vi "LIDAR V9 FPGA Main.vi"() -> ()   [LabVIEW 2013]
uses:
  Controls/FPGA Nain State.ctl
  Controls/Scan Format Typedaf.ctl
  <vilib>/Platform/TimedLoop/XDataNode/timing_clust.ctl
  <vilib>/Platform/TimedLoop/XDataNode/nitl_modes.ctl
  <vilib>/Platform/TimedLoop/XDataNode/wakeup.ctl
  Controls/Algorithm State.ctl
  <vilib>/rvi/Emulation/niFpgaSctlEmulationGetInTimedLoop.vi
  <vilib>/rvi/DataTransferAndStorage/Container/Common/niFpgaContainerGetUniqueNameForEmu.vi
  <vilib>/rvi/DataTransferAndStorage/Container/Common/niFpgaContainerSetEmuInfo.vi
  <vilib>/rvi/eio/common/nirviEmuReportErrorAndStop.vi
  <vilib>/rvi/Emulation/niFpgaEmulationReportErrorSimple.vi
  <vilib>/rvi/Emulation/niFpgaGetClockAttributes.vi
  <vilib>/rvi/Emulation/niFpgaCriticalErrorInLSC.vi
  <vilib>/rvi/eio/common/nirviEmuTemplateMethod_errors.vi
  <vilib>/rvi/FIFO/Fifo_Resource/nirvififoEmulationWriteFpgaImpl.vi
  <vilib>/rvi/DataTransferAndStorage/Container/Common/niFpgaContainerExecOnDevCompGetState.vi
  <vilib>/rvi/DataTransferAndStorage/Register/Emulation/niFpgaRegisterEmulationFpgaImpl.vi
  <instcachedir>/0/niFpgaRegisterEmulationFpgaImpl_DCF4BC0110594B98B44A971D60CEEC4D.lvgen/niFpgaRegisterEmulationFpgaImpl_DCF4BC0110594B98B44A971D60CEEC4D_000.vi
  <vilib>/rvi/FIFO/Fifo_Resource/nirvififoEmulationReadFpgaImpl.vi
  LIDAR V2 Globals.vi
  <vilib>/rvi/Emulation/niFpgaProcessEmulError.vi
  <vilib>/rvi/interface/RandomDataEmulation/nirviRandomDataFPGAFIFO.vi
  <vilib>/rvi/interface/RandomDataEmulation/niFpgaRandomDataHandleErrors.vi
  <vilib>/Platform/TimedLoop/XDataNode/XDataNode.xnode
  <vilib>/rvi/LocalResourceManager/LocalResourceManager.xnode
  <vilib>/eio/EIONode/EIONode.xnode
  <vilib>/rvi/DataTransferAndStorage/Container/XNode/niFpgaContainer.xnode
  <vilib>/rvi/FIFO/Fifo_Resource/nirvififoEmulationWrite.vi
  <vilib>/rvi/DataTransferAndStorage/Register/Emulation/niFpgaRegisterEmulationRefIn.vi
  <vilib>/rvi/FIFO/Fifo_Resource/nirvififoEmulationRead.vi
  <vilib>/rvi/interface/RandomDataEmulation/nirviRandomDataFpgaReadWriteTemplate.vi
  <vilib>/Platform/TimedLoop/XDataNode/XDNodeRunTimeDep.lvlib
panel:
  in  "MaxStartSample":u8
  in  "LedScanDebEn":bool
  in  "ActiveLedIndexDeb":u16
  in  "10thIndexDeb":u8
  in  "PulseUpClck":u16=3
  in  "PulseWaitClck":u16=40
  in  "Devider":u8=3
  in  "PFI3":bool
  in  "PFI2":bool
  in  "User Command Commit":bool
  in  "User Command":u8
  out "User Command Idle":bool
  out "User Command Status":u8
  in  "User Data 0":u8
  in  "User Data 1":u8
  out "User Error":bool
  out "Configured?":bool
  in  "MemDebStart":u32
  in  "MemDebEnd":u32
  in  "ReadMemSel":bool
  in  "ReadMem":bool
  in  "NextLedEn":bool
  out "SimOut":i16
  out "PLL Locked":bool
  out "LedAddress":u16
  in  "SingleCycle":bool
  in  "PulsePerLed":i16=199
  in  "ScanFormat":T1=enum."FullScanPerLed"
  in  "SamplingEnable":bool
  out "MainState":T2
  out "10thIndex":u8
  out "PulseIndex":i16
  in  "MemSel":bool
  in  "ActiveLedIndex":u16
  out "InitMem":bool
  out "PulseEnd":bool
  in  "SampPerPulse":u16=99
  out "IterReset":u16 format="%.0b"
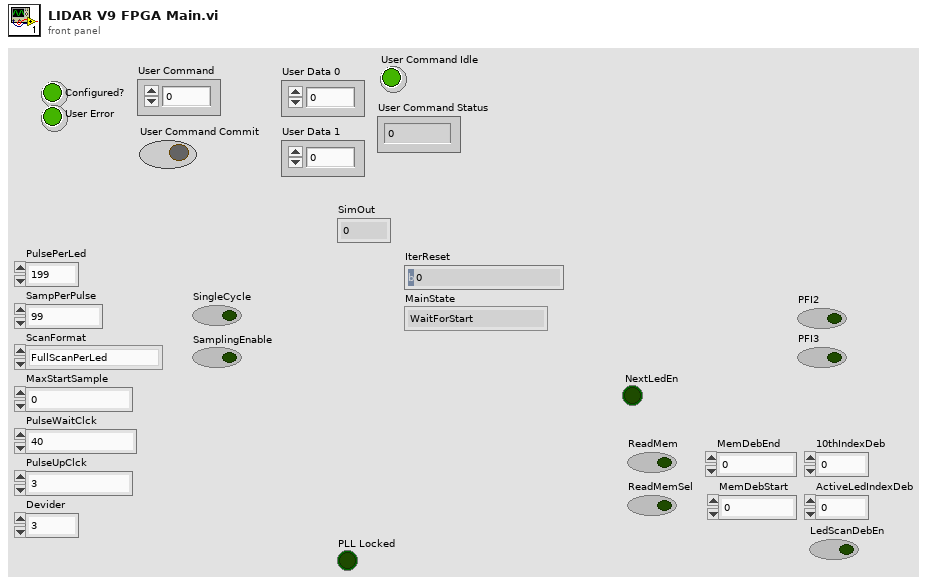
[diagram p1: front panel]
types:
  T1 = typedef "Scan Format Typedaf.ctl" = enum16{"1PulsePerLed", "FullScanPerLed"}
  T2 = typedef "FPGA Nain State.ctl" = enum16{"WaitForStart", "SetProcParams", "SelectActiveLed", "ActivatePulse", "WaitForPulseEnd", "WaitForAlgoStart", "SingleCycleEnd"}
  T3 = typedef "XDNodeRunTimeDep.lvlib/timing_clust.ctl" = cluster{"Expected End [f-1]":u64, "Actual End [f-1]":u64, "Finished Late? [f-1]":bool, "Expected End [i-1]":u64, "Actual End [i-1]":u64, "Finished Late? [i-1]":bool, "Expected Start [i]":u64, "Actual Start [i]":u64, "Expected Start [f]":u64, "Actual Start [f]":u64, "Source Name":string, "Structure Name":string, "Period":i64, "Deadline":i64, "Offset":i64, "Start":i64, "Priority":i32, "Timeout":i32, "Mode":T4, "Wakeup Reason":T5, "Error":errorcluster, "Source Type":string, "Secondary Source Type":string, "Global End Time":u64, "Global Start Time":u64, "Frame Duration":u64, "Iteration Duration":u64, "Assigned CPU":i32, "I/O Scan Engine Mode":u32}
  T4 = typedef "XDNodeRunTimeDep.lvlib/nitl_modes.ctl" = enum32{"No Change", "Process missed periods, maintain original phase", "Discard missed periods, maintain original phase", "Process missed periods, ignore original phase", "Discard missed periods, ignore original phase"}
  T5 = typedef "XDNodeRunTimeDep.lvlib/wakeup.ctl" = enum32{"Normal", "Aborted", "Asynchronous wakeup", "Timing source error", "Timed loop error", "Timeout"}
  T6 = typedef "Algorithm State.ctl" = enum16{"WaitForStart", "GetNextSignalElement", "WaitForNextSignalElem", "MultWithSinc", "CalcMax"}
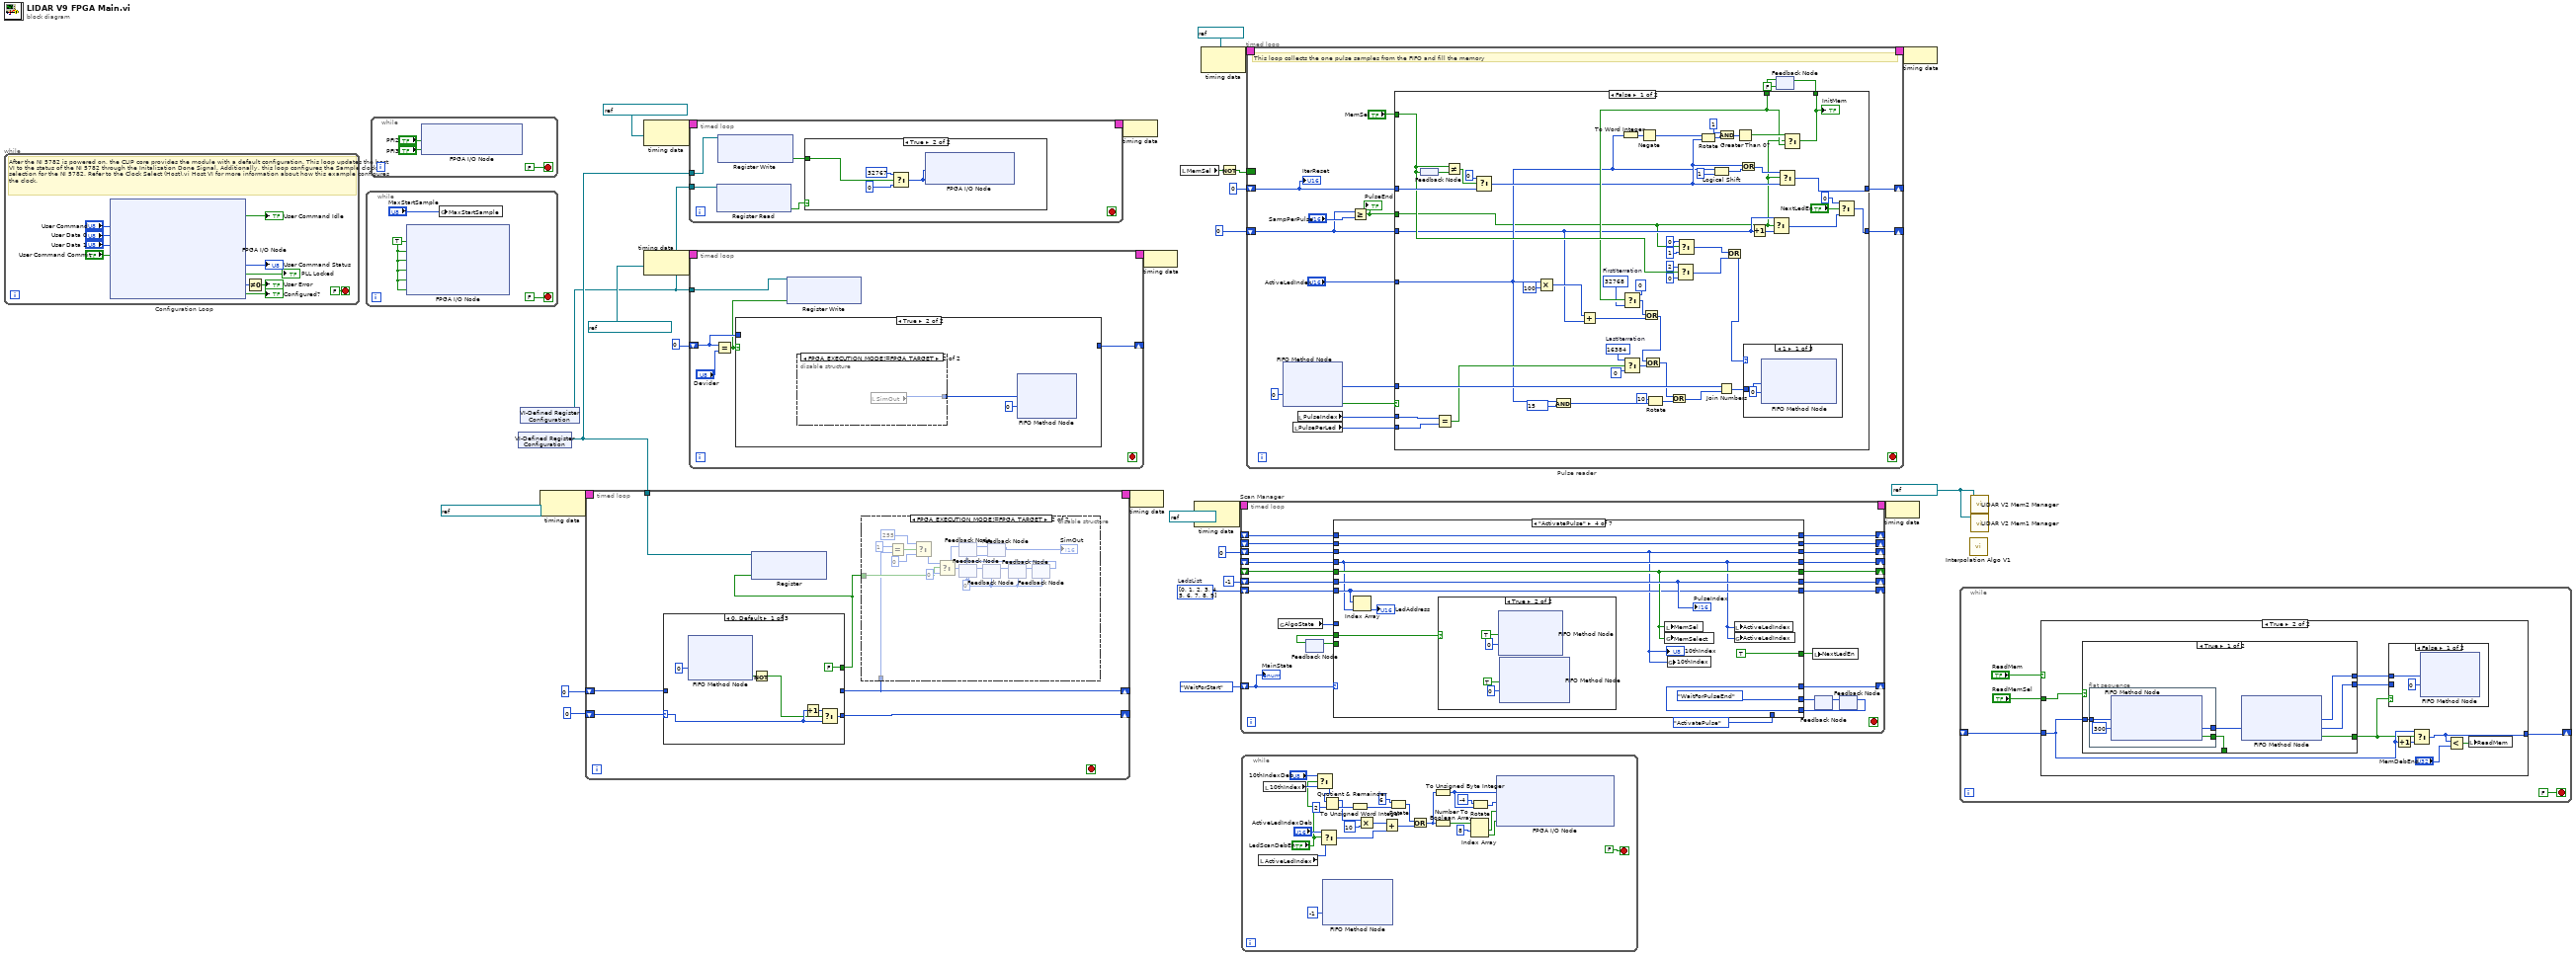
[diagram p0: block diagram]
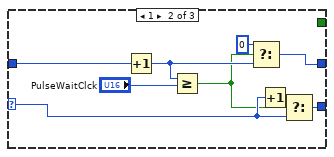
[diagram p4: hidden frame]
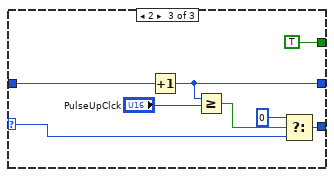
[diagram p5: hidden frame]
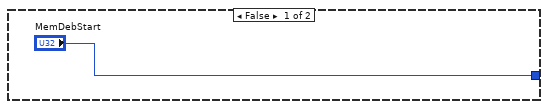
[diagram p6: hidden frame]
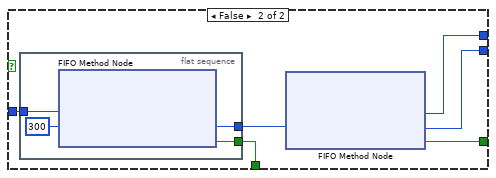
[diagram p8: hidden frame]
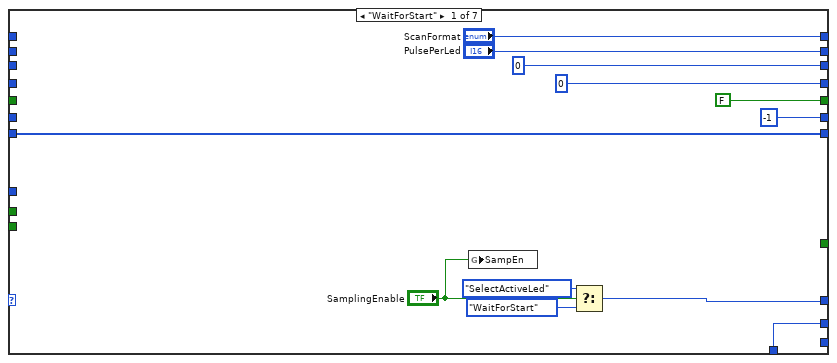
[diagram p9: hidden frame]
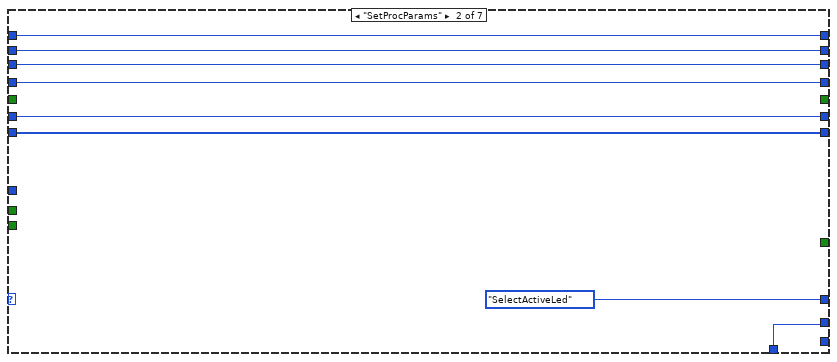
[diagram p10: hidden frame]
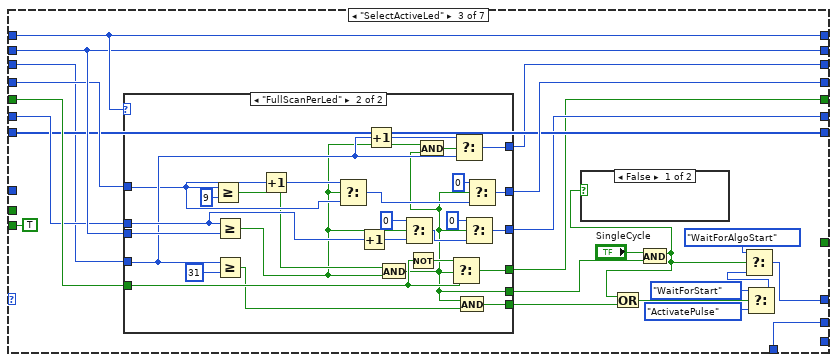
[diagram p11: hidden frame]
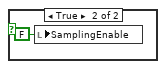
[diagram p12: hidden frame]
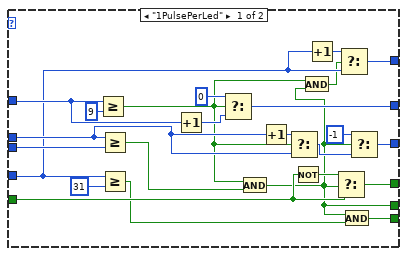
[diagram p13: hidden frame]
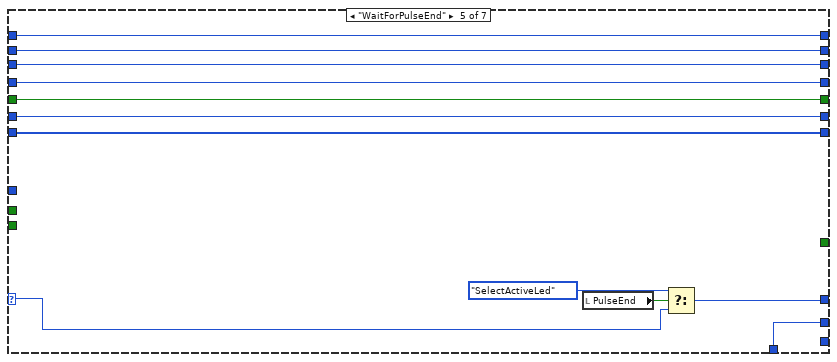
[diagram p15: hidden frame]
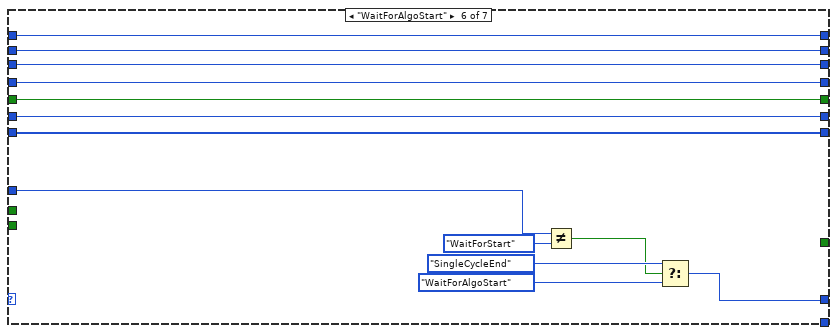
[diagram p16: hidden frame]
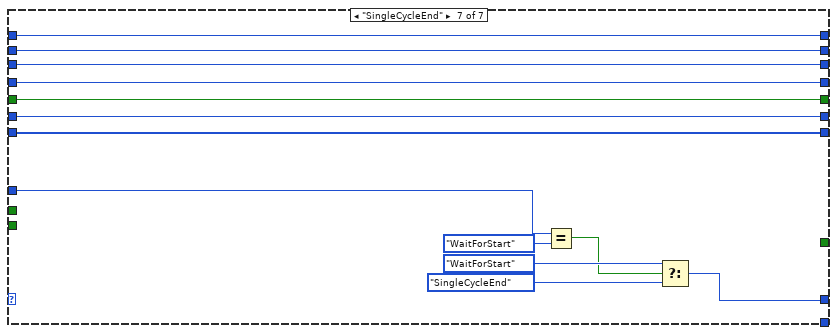
[diagram p17: hidden frame]
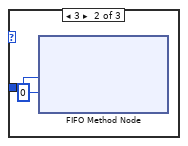
[diagram p18: hidden frame]
diagram:
  w1 = refnum<k21> "83.33MHz" ("Source Name")
  w17 = u16[] [0, 1, 2, 3, 4, 5, 6, 7, 8, 9]  # LedsList
  n1 = while "Configuration Loop" {
    stop <- FALSE stop-if-true
    # "After the NI 5782 is powered on, the CLIP core provides the module with a default configuration. This loop updates the host VI to the status of the NI 5782 through the Initalization Done Signal. Additionally, this loop configures the Sample clock selection for the NI 5782. Refer to the Clock Select (Host).vi Host VI for more information about how this example configures the clock."
    n2 = xnode "FPGA I/O Node"("IO Module\\User Command"="User Command", "IO Module\\User Data 0"="User Data 0", "IO Module\\User Data 1"="User Data 1", "IO Module\\User Command Commit"="User Command Commit") -> ("IO Module\\User Command Idle"=→"User Command Idle":bool, "IO Module\\User Command Status"=→"User Command Status":u8, "IO Module\\PLL Locked"=→"PLL Locked":bool, "IO Module\\User Error"=w34:u8, "IO Module\\Initialization Done"=→"Configured?":bool)  [unwired: 9 in, 9 out]
    n3 = Not Equal To 0?(x=w34) -> (x != 0?=→"User Error":bool)
  }
  n4 = while {
    stop <- FALSE stop-if-true
    w42 = TRUE ("IO Module\\DIO Port 0 WE")
    n5 = xnode "FPGA I/O Node"("IO Module\\DIO Port 0 WE"=w42, "IO Module\\DIO Port 1 WE"=w42, "IO Module\\PFI 0 WE"=w42, "IO Module\\PFI 1 WE"=w42, "IO Module\\PFI 2 WE"=w42, "IO Module\\PFI 3 WE"=w42) -> ()  [unwired: 6 in, 6 out]
    n6 = global write "LIDAR V2 Globals.vi" "MaxStartSample"("MaxStartSample") -> ()
  }
  n7 = while {
    stop <- FALSE stop-if-true
    n8 = xnode "FPGA I/O Node"("IO Module\\PFI 2 Wr Data"="PFI2", "IO Module\\PFI 3 Wr Data"="PFI3") -> ()  [unwired: 2 in, 2 out]
  }
  n9 = xnode ("VI-Defined Register Configuration")() -> ("Register Out"=w3:refnum<k21>)
  n10 = xnode ("VI-Defined Register Configuration")() -> ("Register Out"=w2:refnum<k21>)
  n11 = node-c288(refnum<k21> "IO Module\\Data Clock Div 2" ("Source Name")) -> (w11:T3)
  n12 = timed-loop {
    timing: w11 -> [_]
    timing-out: [_] -> w10
    shift-right: [w51] -> _
    shift-left: i16 0 -> [w52]
    shift-right: [w49] -> _
    shift-left: u16 0 -> [w50]
    tunnel: w3 -> [w48]
    stop <- _ stop-if-true
    n13 = case shown="0, Default" w52 {
      selector: w52 -> [w74 w81 w87]
      tunnel: [w75 w82 w88] -> w51
      tunnel: w50 -> [_ w84 w92]
      tunnel: [_ w78 w91] -> w49
      tunnel: [FALSE _ TRUE] -> w47
      frame 0, Default {
        n14 = xnode ("FIFO Method Node")("Timeout"=0) -> ("Timed Out?"=w71:bool)  [unwired: 1 in, 2 out]
        n15 = Not(x=w71) -> (.not. x?=w69:bool)
        n16 = Increment(x=w74) -> (x+1=w73:i16)
        n17 = Select(t=w73, s=w69, f=w74) -> (s? t:f=w75:i16)
      }
      frame 1 {
        n18 = Increment(x=w84) -> (x+1=w79:u16)
        n19 = Greater Or Equal?(x=w79, y="PulseWaitClck") -> (x >= y?=w76:bool)
        n20 = Select(t=u16 0, s=w76, f=w79) -> (s? t:f=w78:u16)
        n21 = Increment(x=w81) -> (x+1=w80:i16)
        n22 = Select(t=w80, s=w76, f=w81) -> (s? t:f=w82:i16)
      }
      frame 2 {
        n23 = Increment(x=w92) -> (x+1=w91:u16)
        n24 = Greater Or Equal?(x=w91, y="PulseUpClck") -> (x >= y?=w89:bool)
        n25 = Select(t=i16 0, s=w89, f=w87) -> (s? t:f=w88:i16)
      }
    }
    n26 = xnode "Register"("Data"=w47, "Register In"=w48) -> ()  [unwired: 1 out]
    n27 = disable-structure shown="FPGA_EXECUTION_MODE!=FPGA_TARGET" {
      disable-tunnel: w47 -> [_ w60]
      disable-tunnel: w49 -> [_ w59]
      frame condition #0 (active) {
      }
      frame condition #1 {
        w63 = i16 0 ("IO Module\\AO 0")
        n28 = Equal?(x=u16 1, y=w59) -> (x = y?=w57:bool)
        n29 = Select(t=i16 255 ("IO Module\\AO 0"), s=w57, f=i16 0) -> (s? t:f=w58:i16)
        n30 = Select(t=w58, s=w60, f=i16 0 ("IO Module\\AO 0")) -> (s? t:f=w61:i16)
        n31 = feedback-in #1(w61) -> ()
        n32 = feedback #1(w63) -> (w68:i16)
        n33 = feedback #2(w63) -> (w64:i16)
        n34 = feedback #3(w63) -> (w67:i16)
        n35 = feedback-in #3(w68) -> ()
        n36 = feedback #4(w63) -> (→"SimOut":i16)
        n37 = feedback-in #4(w64) -> ()
        n38 = feedback #5(w63) -> (w66:i16)
        n39 = feedback-in #5(w67) -> ()
        n40 = feedback #6(w63) -> (w65:i16)
        n41 = feedback-in #2(w65) -> ()
        n42 = feedback-in #6(w66) -> ()
      }
    }
  }
  n43 = node-c288(refnum<k21> "IO Module\\Data Clock" ("Source Name")) -> (w6:T3)
  n44 = node-c288(refnum<k21> "IO Module\\Data Clock" ("Source Name")) -> (w29:T3)
  n45 = timed-loop {
    timing: w6 -> [_]
    timing-out: [_] -> w5
    tunnel: w3 -> [w98]
    tunnel: w2 -> [w96]
    stop <- _ stop-if-true
    n46 = xnode "Register Read"("Register In"=w96) -> ("Data"=w95:bool)  [unwired: 1 out]
    n47 = xnode "Register Write"("Register In"=w98) -> ("Data"=w97:bool)  [unwired: 1 out]
    n48 = case shown="True" w95 {
      tunnel: w97 -> [_ w99]
      frame False {
      }
      frame True {
        n49 = Select(t=i16 32767 ("IO Module\\AO 0"), s=w99, f=i16 0 ("IO Module\\AO 0")) -> (s? t:f=w100:i16)
        n50 = xnode "FPGA I/O Node"("IO Module\\AO 0 N-1"=w100, "IO Module\\AO 0 N"=w100) -> ()  [unwired: 2 in, 2 out]
      }
    }
  }
  n51 = timed-loop {
    timing: w29 -> [_]
    timing-out: [_] -> w28
    shift-right: [w107] -> _
    shift-left: u8 0 -> [w108]
    tunnel: w2 -> [w106]
    stop <- _ stop-if-true
    n52 = Equal?(x=w108, y="Devider") -> (x = y?=w105:bool)
    n53 = case shown="True" w105 {
      tunnel: w108 -> [w111 _]
      tunnel: [w110 _] -> w107
      frame False {
        n54 = Increment(x=w111) -> (x+1=w110:u8)
      }
      frame True {
        n55 = disable-structure shown="FPGA_EXECUTION_MODE!=FPGA_TARGET" {
          disable-tunnel: [w114 w115] -> w112
          frame condition #0 (active) {
            n56 = xnode "FPGA I/O Node"() -> ("IO Module\\AI 0"=w114:i16)  [unwired: 1 in, 1 out]
          }
          frame condition #1 {
            n57 = local read "SimOut"() -> (w115:i16)
          }
        }
        n58 = xnode ("FIFO Method Node")("Element"=w112, "Timeout"=0) -> ()  [unwired: 1 in, 2 out]
      }
    }
    n59 = xnode "Register Write"("Data"=w105, "Register In"=w106) -> ()  [unwired: 1 out]
  }
  n60 = node-c288(w5) -> ()
  n61 = node-c288(w10) -> ()
  n62 = node-c288(w28) -> ()
  n63 = local read "MemSel"() -> (w22:bool)
  n64 = node-c288(refnum<k21> "83.33MHz" ("Source Name")) -> (w25:T3)
  n65 = node-c288(refnum<k21> "83.33MHz" ("Source Name")) -> (w27:T3)
  n66 = Not(x=w22) -> (.not. x?=w21:bool)
  n67 = timed-loop "Scan Manager" {
    timing: w25 -> [_]
    timing-out: [_] -> w24
    shift-right: [w140] -> _
    shift-left: FPGA_Nain_State."WaitForStart" ("MainState") -> [w141]
    shift-right: [w139] -> _
    shift-left: _ -> [w137]
    shift-right: [w138] -> _
    shift-left: _ -> [w136]
    shift-right: [w129] -> _
    shift-left: u8 0 ("10thIndex") -> [w135]
    shift-right: [w119] -> _
    shift-left: _ -> [w134]
    shift-right: [w123] -> _
    shift-left: _ -> [w133]
    shift-right: [w132] -> _
    shift-left: i16 -1 -> [w122]
    shift-right: [w130] -> _
    shift-left: w17 -> [w131]
    stop <- _ stop-if-true
    n68 = global read "LIDAR V2 Globals.vi" "AlgoState"() -> (w118:T6)
    n69 = feedback #7() -> (w120:bool)  [unwired: 1 in]
    n70 = feedback #8() -> (w126:T2)  [unwired: 1 in]
    n71 = feedback #9() -> (w125:T2)  [unwired: 1 in]
    n72 = case shown="\"ActivatePulse\"" w141 {
      selector: w141 -> [_ _ _ _ w257 _ _]
      tunnel: [w151 FPGA_Nain_State."SelectActiveLed" ("MainState") w165 w243 w256 w267 w280] -> w140
      tunnel: ["ScanFormat" w157 w184 w247 w263 w276 w289] -> w139
      tunnel: ["PulsePerLed" w156 w182 w246 w262 w275 w288] -> w138
      tunnel: w137 -> [_ w157 w184 w247 w263 w276 w289]
      tunnel: w136 -> [_ w156 w182 w246 w262 w275 w288]
      tunnel: [u8 0 ("10thIndex") w155 w173 w236 w261 w274 w287] -> w129
      tunnel: w135 -> [_ w155 w174 w236 w261 w274 w287]
      tunnel: [u16 0 ("ActiveLedIndex") w154 w179 w237 w260 w273 w286] -> w119
      tunnel: w134 -> [_ w154 w180 w237 w260 w273 w286]
      tunnel: [FALSE _ w176 w240 w259 w272 w285] -> w123
      tunnel: w133 -> [_ _ w183 w240 w259 w272 w285]
      tunnel: [i16 -1 ("t") w160 w177 w241 w254 w271 w284] -> w132
      tunnel: w122 -> [_ w160 w181 w241 w254 w271 w284]
      tunnel: w131 -> [w149 w159 w178 w238 w253 w270 w283]
      tunnel: [w149 w159 w178 w238 w253 w270 w283] -> w130
      tunnel: [_ _ _ TRUE ("SampEnable") _ _ _] -> w128
      tunnel: [w148 w158 w172 FPGA_Nain_State."WaitForPulseEnd" ("MainState") w252 _ _] -> w127
      tunnel: w125 -> [_ _ _ w243 _ _ _]
      tunnel: FPGA_Nain_State."ActivatePulse" ("MainState") -> [w148 w158 w172 _ w252 _ _]
      tunnel: [_ _ TRUE _ _ _ _] -> w121
      tunnel: w120 -> [_ _ _ w242 _ _ _]
      tunnel: w118 -> [_ _ _ _ _ w264 w278]
      frame "WaitForStart" {
        n73 = global write "LIDAR V2 Globals.vi" "SampEn"("SamplingEnable") -> ()
        n74 = Select(t=FPGA_Nain_State."SelectActiveLed" ("MainState"), s="SamplingEnable", f=FPGA_Nain_State."WaitForStart" ("MainState")) -> (s? t:f=w151:T2)
      }
      frame "SetProcParams" {
      }
      frame "SelectActiveLed" {
        n75 = case shown="\"FullScanPerLed\"" w184 {
          tunnel: w183 -> [w201 w231]
          tunnel: w174 -> [w194 w226]
          tunnel: w182 -> [w204 w233]
          tunnel: w180 -> [w207 w217]
          tunnel: w181 -> [w203 w232]
          tunnel: [w195 w213] -> w179
          tunnel: [w190 w215] -> w177
          tunnel: [w198 w229] -> w176
          tunnel: [w196 w227] -> w170
          tunnel: [w192 w224] -> w173
          tunnel: [w186 w210] -> w171
          frame "1PulsePerLed" {
            n76 = Greater Or Equal?(x=w207, y=u16 9) -> (x >= y?=w188:bool)
            n77 = Greater Or Equal?(x=w203, y=w204) -> (x >= y?=w199:bool)
            n78 = Greater Or Equal?(x=w194, y=u8 31) -> (x >= y?=w197:bool)
            n79 = Increment(x=w207) -> (x+1=w206:u16)
            n80 = Select(t=u16 0, s=w188, f=w206) -> (s? t:f=w195:u16)
            n81 = And(x=w188, y=w199) -> (x .and. y?=w186:bool)
            n82 = Increment(x=w203) -> (x+1=w202:i16)
            n83 = Select(t=w202, s=w188, f=w203) -> (s? t:f=w191:i16)
            n84 = Not(x=w201) -> (.not. x?=w200:bool)
            n85 = And(x=w188, y=w186) -> (x .and. y?=w187:bool)
            n86 = Increment(x=w194) -> (x+1=w193:u8)
            n87 = Select(t=w200, s=w186, f=w201) -> (s? t:f=w198:bool)
            n88 = Select(t=w193, s=w187, f=w194) -> (s? t:f=w192:u8)
            n89 = And(x=w186, y=w197) -> (x .and. y?=w196:bool)
            n90 = Select(t=i16 -1, s=w186, f=w191) -> (s? t:f=w190:i16)
          }
          frame "FullScanPerLed" {
            n91 = Greater Or Equal?(x=w217, y=u16 9) -> (x >= y?=w216:bool)
            n92 = Greater Or Equal?(x=w232, y=w233) -> (x >= y?=w211:bool)
            n93 = Greater Or Equal?(x=w226, y=u8 31) -> (x >= y?=w228:bool)
            n94 = Increment(x=w217) -> (x+1=w218:u16)
            n95 = Select(t=w218, s=w211, f=w217) -> (s? t:f=w214:u16)
            n96 = Increment(x=w232) -> (x+1=w220:i16)
            n97 = Increment(x=w226) -> (x+1=w225:u8)
            n98 = And(x=w216, y=w211) -> (x .and. y?=w210:bool)
            n99 = Select(t=i16 0, s=w211, f=w220) -> (s? t:f=w223:i16)
            n100 = Not(x=w231) -> (.not. x?=w230:bool)
            n101 = And(x=w211, y=w210) -> (x .and. y?=w221:bool)
            n102 = Select(t=w230, s=w210, f=w231) -> (s? t:f=w229:bool)
            n103 = Select(t=w225, s=w221, f=w226) -> (s? t:f=w224:u8)
            n104 = And(x=w210, y=w228) -> (x .and. y?=w227:bool)
            n105 = Select(t=i16 0, s=w210, f=w223) -> (s? t:f=w215:i16)
            n106 = Select(t=u16 0, s=w210, f=w214) -> (s? t:f=w213:u16)
          }
        }
        n107 = And(x="SingleCycle", y=w171) -> (x .and. y?=w162:bool)
        n108 = case shown="False" w162 {
          frame False {
          }
          frame True {
            n109 = local write "SamplingEnable"(FALSE ("SamplingEnable")) -> ()
          }
        }
        n110 = Or(x=w162, y=w170) -> (x .or. y?=w169:bool)
        n111 = Select(t=FPGA_Nain_State."WaitForStart" ("MainState"), s=w169, f=FPGA_Nain_State."ActivatePulse" ("MainState")) -> (s? t:f=w166:T2)
        n112 = Select(t=FPGA_Nain_State."WaitForAlgoStart" ("MainState"), s=w162, f=w166) -> (s? t:f=w165:T2)
      }
      frame "ActivatePulse" {
        n113 = Index Array(array=w238, index=w237) -> (element=→"LedAddress":u16)
        n114 = case shown="True" w242 {
          frame False {
          }
          frame True {
            n115 = xnode ("FIFO Method Node")("Element"=TRUE ("GenPulse"), "Timeout"=0) -> ()  [unwired: 1 in, 2 out]
            n116 = xnode ("FIFO Method Node")("Element"=TRUE ("GenPulse"), "Timeout"=0) -> ()  [unwired: 1 in, 2 out]
          }
        }
        n117 = local write "MemSel"(w240) -> ()
        n118 = global write "LIDAR V2 Globals.vi" "MemSelect"(w240) -> ()
        n119 = global write "LIDAR V2 Globals.vi" "10thIndex"(w236) -> ()
        n120 = local write "ActiveLedIndex"(w237) -> ()
        n121 = global write "LIDAR V2 Globals.vi" "ActiveLedIndex"(w237) -> ()
        "PulseIndex" <- w241
        "10thIndex" <- w236
      }
      frame "WaitForPulseEnd" {
        n122 = local read "PulseEnd"() -> (w258:bool)
        n123 = Select(t=FPGA_Nain_State."SelectActiveLed", s=w258, f=w257) -> (s? t:f=w256:T2)
      }
      frame "WaitForAlgoStart" {
        n124 = Not Equal?(x=w264, y=Algorithm_State."WaitForStart") -> (x != y?=w265:bool)
        n125 = Select(t=FPGA_Nain_State."SingleCycleEnd", s=w265, f=FPGA_Nain_State."WaitForAlgoStart" ("MainState")) -> (s? t:f=w267:T2)
      }
      frame "SingleCycleEnd" {
        n126 = Equal?(x=w278, y=Algorithm_State."WaitForStart") -> (x = y?=w277:bool)
        n127 = Select(t=FPGA_Nain_State."WaitForStart", s=w277, f=FPGA_Nain_State."SingleCycleEnd" ("MainState")) -> (s? t:f=w280:T2)
      }
    }
    n128 = feedback-in #7(w121) -> ()
    n129 = local write "NextLedEn"(w128) -> ()
    n130 = feedback-in #8(w127) -> ()
    n131 = feedback-in #9(w126) -> ()
    "MainState" <- w141
  }
  n132 = while {
    stop <- FALSE stop-if-true
    n133 = local read "ActiveLedIndex"() -> (w296:u16)
    n134 = local read "10thIndex"() -> (w298:u8)
    n135 = Select(t="10thIndexDeb", s="LedScanDebEn", f=w298) -> (s? t:f=w297:u8)
    n136 = Select(t="ActiveLedIndexDeb", s="LedScanDebEn", f=w296) -> (s? t:f=w295:u16)
    n137 = xnode ("FIFO Method Node")("Timeout"=-1) -> ()  [unwired: 1 in, 3 out]
    n138 = Quotient & Remainder(x=w297, y=u8 2) -> (x-y*floor(x/y)=w302:u8, floor(x/y)=w303:u8)
    n139 = To Unsigned Word Integer(number=w303) -> (unsigned 16bit integer=w310:u16)
    n140 = Multiply(x=w302, y=u8 10) -> (x*y=w301:u8)
    n141 = Add(x=w301, y=w295) -> (x+y=w316:u16)
    n142 = Rotate(1:w310, 2:u16 6 ("x")) -> (0:w317:u16)
    n143 = Or(x=w317, y=w316) -> (x .or. y?=w315:u16)
    n144 = To Unsigned Byte Integer(number=w315) -> (unsigned 8bit integer=w307:u8)
    n145 = Number To Boolean Array(number=w315) -> (Boolean array=w314:bool[])
    n146 = Index Array(array=w314, index #1=8 ("index")) -> (element #1=w312:bool, element #2=w311:bool)  [unwired: 1 in]
    n147 = Rotate(1:w307, 2:i16 -4 ("y")) -> (0:w305:u8)
    n148 = xnode "FPGA I/O Node"("IO Module\\DIO Port 0 Wr Data"=w307, "IO Module\\DIO Port 1 Wr Data"=w305, "IO Module\\PFI 0 Wr Data"=w312, "IO Module\\PFI 1 Wr Data"=w311) -> ()  [unwired: 4 in, 4 out]
  }
  n149 = timed-loop "Pulse reader" {
    timing: w27 -> [_]
    timing-out: [_] -> w26
    shift-right: [w330] -> _
    shift-left: u16 0 -> [w328]
    border: w21 -> [_]
    shift-right: [w321] -> _
    shift-left: u16 0 -> [w319]
    stop <- _ stop-if-true
    # "This loop collects the one pulse samples from the FIFO and fill the memory"
    n150 = xnode ("FIFO Method Node")("Timeout"=0) -> ("Element"=w332:i16, "Timed Out?"=w331:bool)  [unwired: 1 in, 1 out]
    n151 = local read "PulsePerLed"() -> (w322:i16)
    n152 = local read "PulseIndex"() -> (w323:i16)
    n153 = Greater Or Equal?(x=w319, y="SampPerPulse") -> (x >= y?=w318:bool)
    "PulseEnd" <- w318
    n154 = feedback #10(FALSE) -> (w326:bool)
    n155 = case shown="False" w331 {
      tunnel: w332 -> [w383 _]
      tunnel: "ActiveLedIndex" -> [w338 _]
      tunnel: [w363 w394] -> w330
      tunnel: w328 -> [w384 w394]
      tunnel: [w343 w393] -> w327
      tunnel: w326 -> [w342 w393]
      tunnel: "MemSel" -> [w355 _]
      tunnel: w323 -> [w381 _]
      tunnel: w322 -> [w380 _]
      tunnel: [w336 w392] -> w321
      tunnel: w319 -> [w335 w392]
      tunnel: w318 -> [w334 _]
      frame False {
        w373 = u16 16384  # LastIterration
        w340 = u16 32768  # FirstIterration
        n156 = feedback #11() -> (w386:bool)
        n157 = feedback-in #11(w355) -> ()
        n158 = Equal?(x=w381, y=w380) -> (x = y?=w382:bool)
        n159 = Not Equal?(x=w355, y=w386) -> (x != y?=w387:bool)
        n160 = Select(t=u16 0, s=w387, f=w384) -> (s? t:f=w341:u16)
        n161 = Multiply(x=w338, y=u16 100) -> (x*y=w378:u16)
        n162 = And(x=w338, y=u16 15) -> (x .and. y?=w369:u16)
        n163 = Add(x=w378, y=w335) -> (x+y=w377:u16)
        n164 = To Word Integer(number=w338) -> (16bit integer=w349:i16)
        n165 = Select(t=u16 0 ("x"), s=w342, f=w340) -> (s? t:f=w376:u16)
        n166 = Select(t=w373, s=w382, f=u16 0 ("x")) -> (s? t:f=w372:u16)
        n167 = Negate(x=w349) -> (-x=w345:i16)
        n168 = Or(x=w376, y=w377) -> (x .or. y?=w371:u16)
        n169 = Or(x=w371, y=w372) -> (x .or. y?=w366:u16)
        n170 = Rotate(1:w369, 2:i16 10 ("y")) -> (0:w367:u16)
        n171 = Or(x=w366, y=w367) -> (x .or. y?=w365:u16)
        n172 = Select(t=i16 2, s=w355, f=i16 0) -> (s? t:f=w351:i16)
        n173 = Select(t=i16 0, s=w334, f=i16 1) -> (s? t:f=w350:i16)
        n174 = Rotate(1:w341, 2:w345) -> (0:w346:u16)
        n175 = Logical Shift(y=w338, x=u16 1) -> (x << y=w360:u16)
        n176 = Join Numbers(hi=w383, lo=w365) -> ((hi.lo)=w375:u32)
        n177 = And(x=u16 1, y=w346) -> (x .and. y?=w348:u16)
        n178 = Or(x=w350, y=w351) -> (x .or. y?=w352:i16)
        n179 = Greater Than 0?(x=w348) -> (x > 0?=w344:bool)
        n180 = Or(x=w341, y=w360) -> (x .or. y?=w358:u16)
        n181 = case shown="1" w352 {
          tunnel: w375 -> [w388 w390 _]
          frame 1 {
            n182 = xnode ("FIFO Method Node")("Element"=w388, "Timeout"=0) -> ()  [unwired: 1 in, 2 out]
          }
          frame 3 {
            n183 = xnode ("FIFO Method Node")("Element"=w390, "Timeout"=0) -> ()  [unwired: 1 in, 2 out]
          }
          frame Default {
          }
        }
        n184 = Increment(x=w335) -> (x+1=w364:u16)
        n185 = Select(t=w335, s=w334, f=w364) -> (s? t:f=w337:u16)
        n186 = Select(t=w358, s=w334, f=w341) -> (s? t:f=w363:u16)
        n187 = Select(t=w344, s=w334, f=w342) -> (s? t:f=w343:bool)
        "InitMem" <- w343
        n188 = Select(t=u16 0, s="NextLedEn", f=w337) -> (s? t:f=w336:u16)
      }
      frame True {
      }
    }
    n189 = feedback-in #10(w327) -> ()
    "IterReset" <- w328
  }
  n190 = node-c288(w24) -> ()
  n191 = node-c288(w26) -> ()
  n192 = while {
    shift-right: [w399] -> _
    shift-left: _ -> [w398]
    stop <- FALSE stop-if-true
    n193 = case shown="True" "ReadMem" {
      tunnel: "ReadMemSel" -> [_ w406]
      tunnel: ["MemDebStart" w409] -> w399
      tunnel: w398 -> [_ w411]
      frame False {
      }
      frame True {
        n194 = case shown="True" w406 {
          tunnel: w411 -> [w418 w426]
          tunnel: [w417 w425] -> w403
          tunnel: [w416 w424] -> w405
          tunnel: [w415 w423] -> w404
          tunnel: [w414 w422] -> _
          frame True {
            n195 = flat-sequence {
              tunnel: w418 -> [w421]
              tunnel: [w420] -> w415
              tunnel: [w419] -> w414
              frame #0 {
                w420 = 300 ("Timeout")
                n196 = xnode ("FIFO Method Node")("Element"=w421, "Timeout"=w420) -> ("Timed Out?"=w419:bool)  [unwired: 1 in, 1 out]
              }
            }
            n197 = xnode ("FIFO Method Node")("Timeout"=w415) -> ("Element"=w416:u64, "Timed Out?"=w417:bool)  [unwired: 1 in, 1 out]
          }
          frame False {
            n198 = flat-sequence {
              tunnel: w426 -> [w429]
              tunnel: [w428] -> w423
              tunnel: [w427] -> w422
              frame #0 {
                w428 = 300 ("Timeout")
                n199 = xnode ("FIFO Method Node")("Element"=w429, "Timeout"=w428) -> ("Timed Out?"=w427:bool)  [unwired: 1 in, 1 out]
              }
            }
            n200 = xnode ("FIFO Method Node")("Timeout"=w423) -> ("Element"=w424:u64, "Timed Out?"=w425:bool)  [unwired: 1 in, 1 out]
          }
        }
        n201 = case shown="False" w403 {
          tunnel: w405 -> [w413 _]
          tunnel: w404 -> [_ _]
          frame False {
            n202 = xnode ("FIFO Method Node")("Element"=w413, "Timeout"=0) -> ()  [unwired: 1 in, 2 out]
          }
          frame True {
          }
        }
        n203 = Increment(x=w411) -> (x+1=w410:u32)
        n204 = Select(t=w411, s=w403, f=w410) -> (s? t:f=w409:u32)
        n205 = Less?(x=w409, y="MemDebEnd") -> (x < y?=w407:bool)
        n206 = local write "ReadMem"(w407) -> ()
      }
    }
  }
  n207 = call "Interpolation Algo V1.vi"() -> ()  [unwired: 10 in, 2 out]
  n208 = call "LIDAR V2 Mem2 Manager.vi"("Source Name"=w1) -> ()  [unwired: 11 in]
  n209 = call "LIDAR V2 Mem1 Manager.vi"("Source Name"=w1) -> ()  [unwired: 11 in]
